vi "Get Modules.vi"() -> (0 "error out":errorcluster, 1 "FGVs":refnum<vi>[](array[refnum]), 2 "Modules Refs":refnum<vi>[](array[refnum]), 3 "Modules Names":string[](array[string]))   [LabVIEW 2019]
panel:
  in  "Module Name":string
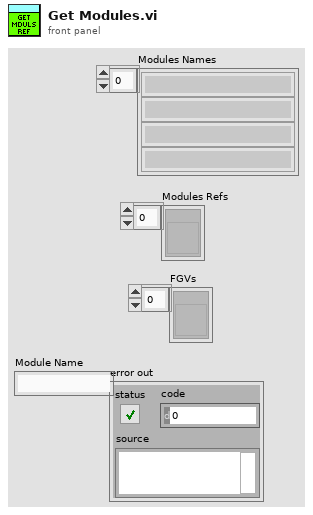
[diagram p1: front panel]
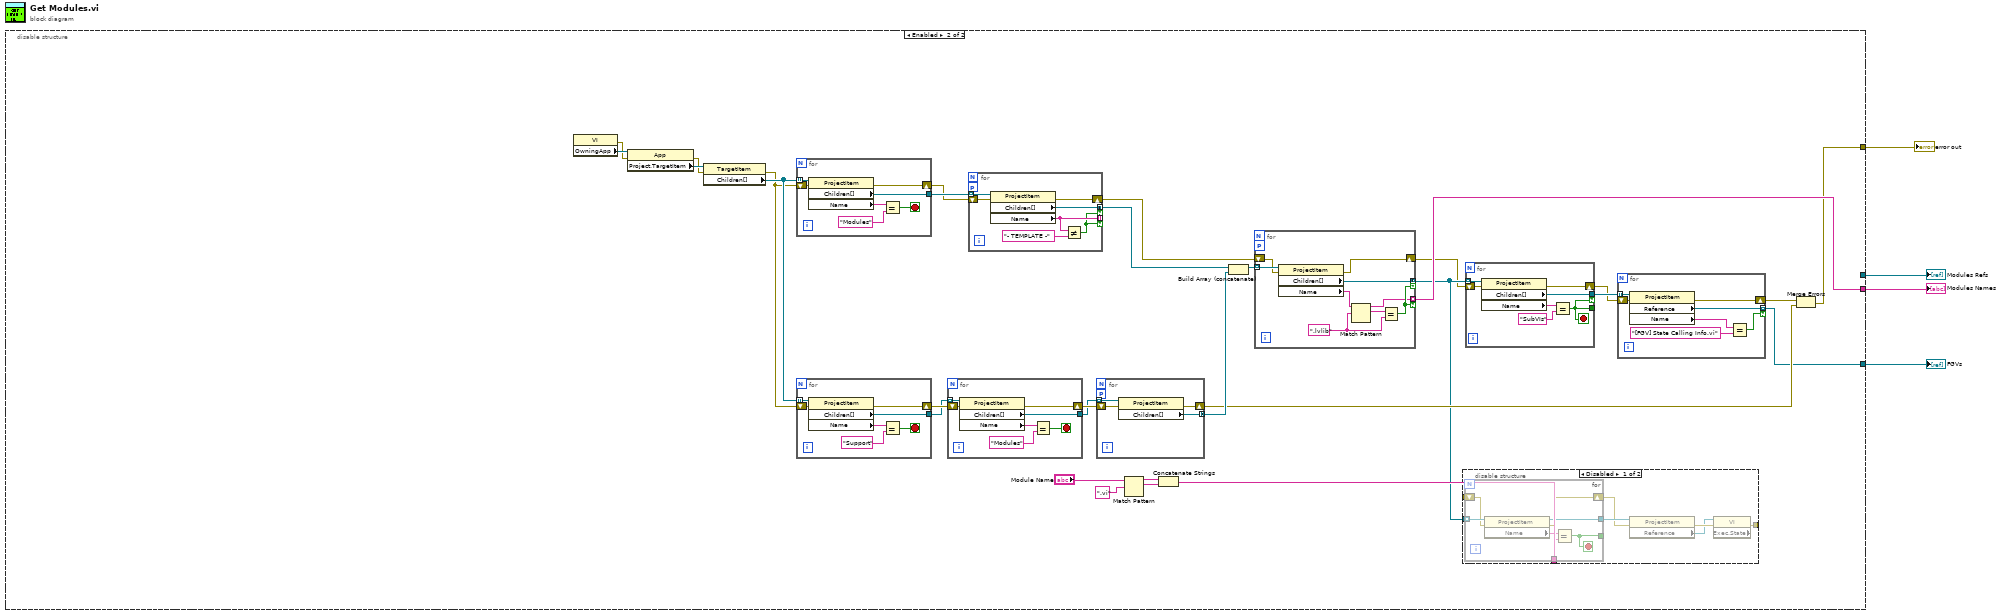
[diagram p0: block diagram]
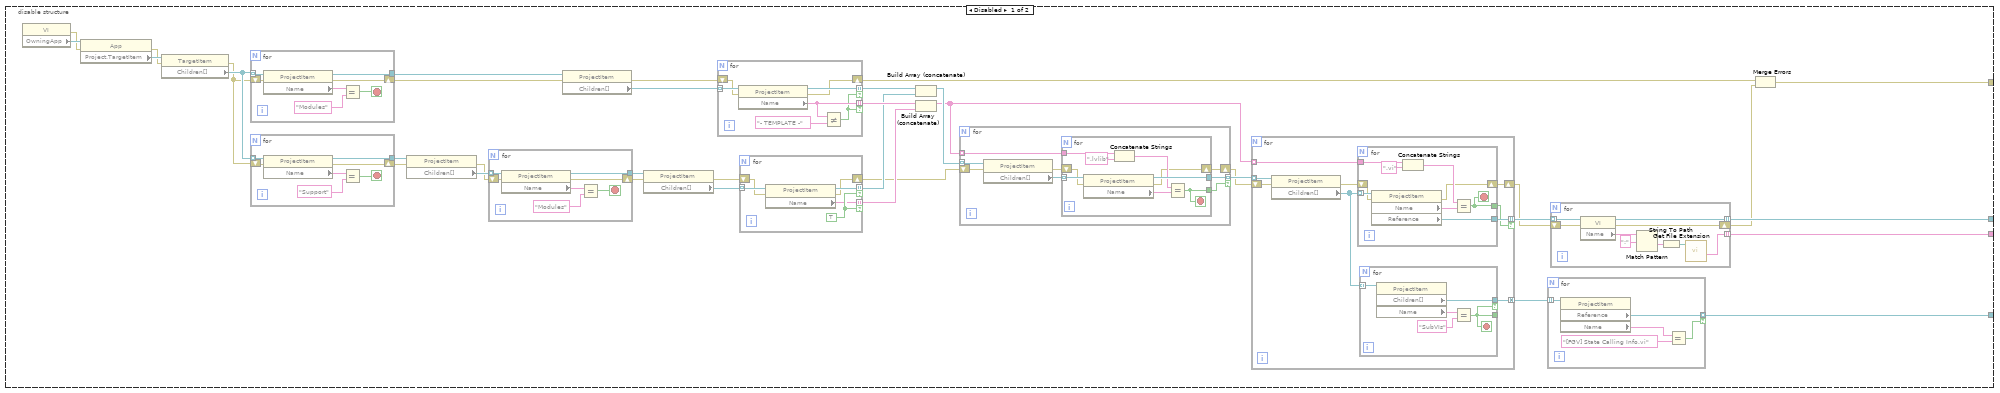
[diagram p2: hidden frame]
diagram:
  n1 = disable-structure shown="Enabled" {
    disable-tunnel: [w23 w142] -> w4
    disable-tunnel: [w22 _] -> w3
    disable-tunnel: [w6 w136] -> w2
    disable-tunnel: [w5 w129] -> w1
    frame Disabled {
      n2 = property class="VI"() -> (error out=w20:errorcluster, "OwningApp"=w36:refnum<vi>)  [unwired: 2 in, 1 out]
      n3 = property class="App"(reference=w36, error in=w20) -> (error out=w19:errorcluster, "Project.TargetItem"=w40:refnum<vi>)  [unwired: 1 out]
      n4 = property class="TargetItem"(reference=w40, error in=w19) -> (error out=w18:errorcluster, "Children[]"=w34:refnum<vi>[])  [unwired: 1 out]
      n5 = for {
        tunnel: w34 -> [w128] mode=indexing
        tunnel: [w124] -> w35
        shift-right: [w122] -> w16
        shift-left: w18 -> [w123]
        stop <- w125 stop-if-true
        n6 = property class="ProjectItem"(reference=w128, error in=w123) -> (reference out=w124:refnum<vi>, error out=w122:errorcluster, "Name"=w127:string)
        n7 = Equal?(x=w127, y="Modules") -> (x = y?=w125:bool)
      }
      n8 = for {
        tunnel: w34 -> [w114] mode=indexing
        tunnel: [w110] -> w33
        shift-right: [w108] -> w17
        shift-left: w18 -> [w109]
        stop <- w111 stop-if-true
        n9 = property class="ProjectItem"(reference=w114, error in=w109) -> (reference out=w110:refnum<vi>, error out=w108:errorcluster, "Name"=w113:string)
        n10 = Equal?(x=w113, y="Support") -> (x = y?=w111:bool)
      }
      n11 = property class="ProjectItem"(reference=w33, error in=w17) -> (error out=w14:errorcluster, "Children[]"=w32:refnum<vi>[])  [unwired: 1 out]
      n12 = for {
        tunnel: w32 -> [w107] mode=indexing
        tunnel: [w103] -> w30
        shift-right: [w101] -> w13
        shift-left: w14 -> [w102]
        stop <- w104 stop-if-true
        n13 = property class="ProjectItem"(reference=w107, error in=w102) -> (reference out=w103:refnum<vi>, error out=w101:errorcluster, "Name"=w106:string)
        n14 = Equal?(x=w106, y="Modules") -> (x = y?=w104:bool)
      }
      n15 = property class="ProjectItem"(reference=w35, error in=w16) -> (error out=w15:errorcluster, "Children[]"=w37:refnum<vi>[])  [unwired: 1 out]
      n16 = property class="ProjectItem"(reference=w30, error in=w13) -> (error out=w12:errorcluster, "Children[]"=w31:refnum<vi>[])  [unwired: 1 out]
      n17 = for {
        tunnel: w37 -> [w120] mode=indexing
        tunnel: [w117] -> w38 mode=indexing if=w118
        tunnel: [w119] -> w39 mode=indexing if=w118
        shift-right: [w115] -> w7
        shift-left: w15 -> [w116]
        n18 = property class="ProjectItem"(reference=w120, error in=w116) -> (reference out=w117:refnum<vi>, error out=w115:errorcluster, "Name"=w119:string)
        n19 = Not Equal?(x=w119, y="- TEMPLATE -") -> (x != y?=w118:bool)
      }
      n20 = for {
        tunnel: w31 -> [w100] mode=indexing
        tunnel: [w97] -> w29 mode=indexing if=w99
        tunnel: [w98] -> w28 mode=indexing if=w99
        shift-right: [w95] -> w11
        shift-left: w12 -> [w96]
        w99 = TRUE
        n21 = property class="ProjectItem"(reference=w100, error in=w96) -> (reference out=w97:refnum<vi>, error out=w95:errorcluster, "Name"=w98:string)
      }
      n22 = Build Array (concatenate)(w38, w29) -> (w27:refnum<vi>[])
      n23 = Build Array (concatenate)(w39, w28) -> (w25:string[])
      n24 = for {
        tunnel: w27 -> [w85] mode=indexing
        tunnel: w25 -> [w84] mode=indexing
        tunnel: [w83] -> w26 mode=indexing if=w82
        shift-right: [w78] -> w10
        shift-left: w11 -> [w80]
        n25 = property class="ProjectItem"(reference=w85, error in=w80) -> (error out=w79:errorcluster, "Children[]"=w81:refnum<vi>[])  [unwired: 1 out]
        n26 = for {
          tunnel: w81 -> [w94] mode=indexing
          tunnel: w84 -> [w93]
          tunnel: [w92] -> w82
          tunnel: [w91] -> w83
          shift-right: [w86] -> w78
          shift-left: w79 -> [w87]
          stop <- w92 stop-if-true
          n27 = property class="ProjectItem"(reference=w94, error in=w87) -> (reference out=w91:refnum<vi>, error out=w86:errorcluster, "Name"=w88:string)
          n28 = Concatenate Strings(w93, ".lvlib" ("string")) -> (w90:string)
          n29 = Equal?(x=w90, y=w88) -> (x = y?=w92:bool)
        }
      }
      n30 = for {
        tunnel: w26 -> [w63] mode=indexing
        tunnel: w25 -> [w62] mode=indexing
        tunnel: [w61] -> w24 mode=indexing if=w60
        tunnel: [w58] -> w21 mode=concatenating
        shift-right: [w55] -> w9
        shift-left: w10 -> [w57]
        n31 = property class="ProjectItem"(reference=w63, error in=w57) -> (error out=w56:errorcluster, "Children[]"=w59:refnum<vi>[])  [unwired: 1 out]
        n32 = for {
          tunnel: w59 -> [w77] mode=indexing
          tunnel: w62 -> [w75]
          tunnel: [w74] -> w60
          tunnel: [w71] -> w61
          shift-right: [w69] -> w55
          shift-left: w56 -> [w70]
          stop <- w74 stop-if-true
          n33 = property class="ProjectItem"(reference=w77, error in=w70) -> (error out=w69:errorcluster, "Name"=w76:string, "Reference"=w71:refnum<vi>)  [unwired: 1 out]
          n34 = Concatenate Strings(w75, ".vi" ("string")) -> (w73:string)
          n35 = Equal?(x=w73, y=w76) -> (x = y?=w74:bool)
        }
        n36 = for {
          tunnel: w59 -> [w68] mode=indexing
          tunnel: [w64] -> _
          tunnel: [w65] -> w58 if=w64
          stop <- w64 stop-if-true
          n37 = property class="ProjectItem"(reference=w68) -> ("Children[]"=w65:refnum<vi>[], "Name"=w66:string)  [unwired: 1 in, 2 out]
          n38 = Equal?(x=w66, y="SubVIs" ("x")) -> (x = y?=w64:bool)
        }
      }
      n39 = for {
        tunnel: w21 -> [w45] mode=indexing
        tunnel: [w42] -> w5 mode=indexing if=w41
        n40 = property class="ProjectItem"(reference=w45) -> ("Reference"=w42:refnum<vi>, "Name"=w43:string)  [unwired: 1 in, 2 out]
        n41 = Equal?(x=w43, y="[FGV] State Calling Info.vi") -> (x = y?=w41:bool)
      }
      n42 = for {
        tunnel: w24 -> [w54] mode=indexing
        tunnel: [w53] -> w22 mode=indexing
        tunnel: [w48] -> w23 mode=indexing
        shift-right: [w46] -> w8
        shift-left: w9 -> [w47]
        n43 = property class="VI"(reference=w54, error in=w47) -> (reference out=w53:refnum<vi>, error out=w46:errorcluster, "Name"=w52:string)
        n44 = Match Pattern(string=w52, regular expression=":") -> (after substring=w50:string)  [unwired: 1 in, 3 out]
        n45 = String To Path(string=w50) -> (path=w49:path)
        n46 = call <vilib>:"Get File Extension.vi"("file"=w49) -> ("filename without extension"=w48:string)  [unwired: 6 in, 4 out]
      }
      n47 = Merge Errors(w7, w8) -> (w6:errorcluster)
    }
    frame Enabled {
      n48 = property class="VI"() -> (error out=w155:errorcluster, "OwningApp"=w156:refnum<vi>)  [unwired: 2 in, 1 out]
      n49 = property class="App"(reference=w156, error in=w155) -> (error out=w154:errorcluster, "Project.TargetItem"=w157:refnum<vi>)  [unwired: 1 out]
      n50 = property class="TargetItem"(reference=w157, error in=w154) -> (error out=w152:errorcluster, "Children[]"=w153:refnum<vi>[])  [unwired: 1 out]
      n51 = for {
        tunnel: w153 -> [w228] mode=indexing
        shift-right: [w224] -> w150
        shift-left: w152 -> [w225]
        tunnel: [w222] -> w151
        stop <- w226 stop-if-true
        n52 = property class="ProjectItem"(reference=w228, error in=w225) -> (error out=w224:errorcluster, "Children[]"=w222:refnum<vi>[], "Name"=w223:string)  [unwired: 1 out]
        n53 = Equal?(x=w223, y="Modules") -> (x = y?=w226:bool)
      }
      n54 = for {
        tunnel: w153 -> [w212] mode=indexing
        shift-right: [w208] -> w158
        shift-left: w152 -> [w209]
        tunnel: [w206] -> w141
        stop <- w210 stop-if-true
        n55 = property class="ProjectItem"(reference=w212, error in=w209) -> (error out=w208:errorcluster, "Children[]"=w206:refnum<vi>[], "Name"=w207:string)  [unwired: 1 out]
        n56 = Equal?(x=w207, y="Support") -> (x = y?=w210:bool)
      }
      n57 = for {
        tunnel: w141 -> [w198] mode=indexing
        shift-right: [w194] -> w140
        shift-left: w158 -> [w195]
        tunnel: [w192] -> w139
        stop <- w196 stop-if-true
        n58 = property class="ProjectItem"(reference=w198, error in=w195) -> (error out=w194:errorcluster, "Children[]"=w192:refnum<vi>[], "Name"=w193:string)  [unwired: 1 out]
        n59 = Equal?(x=w193, y="Modules") -> (x = y?=w196:bool)
      }
      n60 = for {
        tunnel: w151 -> [w205] mode=indexing
        shift-right: [w202] -> w148
        shift-left: w150 -> [w203]
        tunnel: [w201] -> w149 mode=concatenating if=w199
        tunnel: [w200] -> _ mode=indexing if=w199
        workers-P: _ -> [_]
        n61 = property class="ProjectItem"(reference=w205, error in=w203) -> (error out=w202:errorcluster, "Children[]"=w201:refnum<vi>[], "Name"=w200:string)  [unwired: 1 out]
        n62 = Not Equal?(x=w200, y="- TEMPLATE -") -> (x != y?=w199:bool)
      }
      n63 = for {
        tunnel: w139 -> [w191] mode=indexing
        shift-right: [w189] -> w135
        shift-left: w140 -> [w190]
        tunnel: [w188] -> w137 mode=concatenating
        workers-P: _ -> [_]
        n64 = property class="ProjectItem"(reference=w191, error in=w190) -> (error out=w189:errorcluster, "Children[]"=w188:refnum<vi>[])  [unwired: 1 out]
      }
      n65 = Match Pattern(string="Module Name", regular expression=".vi") -> (before substring=w145:string, match substring=w144:string)  [unwired: 1 in, 2 out]
      n66 = Concatenate Strings(w145, w144) -> (w143:string)
      n67 = Build Array (concatenate)(w149, w137) -> (w138:refnum<vi>[])
      n68 = for {
        tunnel: [w218] -> w134 mode=concatenating if=w214
        shift-right: [w221] -> w132
        shift-left: w148 -> [w219]
        tunnel: w138 -> [w220] mode=indexing
        workers-P: _ -> [_]
        tunnel: [w213] -> w142 mode=indexing if=w214
        w215 = ".lvlib" ("string")
        n69 = property class="ProjectItem"(reference=w220, error in=w219) -> (error out=w221:errorcluster, "Children[]"=w218:refnum<vi>[], "Name"=w217:string)  [unwired: 1 out]
        n70 = Match Pattern(string=w217, regular expression=w215) -> (before substring=w213:string, match substring=w216:string)  [unwired: 1 in, 2 out]
        n71 = Equal?(x=w216, y=w215) -> (x = y?=w214:bool)
      }
      n72 = disable-structure shown="Disabled" {
        disable-tunnel: _ -> [w166 _]
        disable-tunnel: w143 -> [w161 _]
        disable-tunnel: [w160 _] -> _
        disable-tunnel: w134 -> [w159 _]
        frame Disabled {
          n73 = for {
            tunnel: w159 -> [w173] mode=indexing
            shift-right: [w171] -> w164
            shift-left: w166 -> [w172]
            tunnel: w161 -> [w169]
            tunnel: [w168] -> w165
            tunnel: [w167] -> _
            stop <- w167 stop-if-true
            n74 = property class="ProjectItem"(reference=w173, error in=w172) -> (reference out=w168:refnum<vi>, error out=w171:errorcluster, "Name"=w170:string)
            n75 = Equal?(x=w170, y=w169) -> (x = y?=w167:bool)
          }
          n76 = property class="ProjectItem"(reference=w165, error in=w164) -> (error out=w163:errorcluster, "Reference"=w162:refnum<vi>)  [unwired: 1 out]
          n77 = property class="VI" props=["Exec.State"](reference=w162, error in=w163) -> (error out=w160:errorcluster)  [unwired: 2 out]
        }
        frame Enabled {
        }
      }
      n78 = for {
        tunnel: w134 -> [w187] mode=indexing
        tunnel: [w183] -> _
        tunnel: [w184] -> w133 if=w183
        shift-right: [w181] -> w131
        shift-left: w132 -> [w182]
        stop <- w183 stop-if-true
        n79 = property class="ProjectItem"(reference=w187, error in=w182) -> (error out=w181:errorcluster, "Children[]"=w184:refnum<vi>[], "Name"=w185:string)  [unwired: 1 out]
        n80 = Equal?(x=w185, y="SubVIs" ("x")) -> (x = y?=w183:bool)
      }
      n81 = for {
        tunnel: w133 -> [w180] mode=indexing
        tunnel: [w177] -> w129 mode=indexing if=w176
        shift-right: [w174] -> w130
        shift-left: w131 -> [w175]
        n82 = property class="ProjectItem"(reference=w180, error in=w175) -> (error out=w174:errorcluster, "Reference"=w177:refnum<vi>, "Name"=w178:string)  [unwired: 1 out]
        n83 = Equal?(x=w178, y="[FGV] State Calling Info.vi") -> (x = y?=w176:bool)
      }
      n84 = Merge Errors(w130, w135) -> (w136:errorcluster)
    }
  }
  "Modules Names" <- w4
  "Modules Refs" <- w3
  "error out" <- w2
  "FGVs" <- w1
